vi "initialize.vi"(0 "HGF_IMAQDevice":refnum<class "HGF_ImaqFg.lvclass">, 3 "initializationData":variant, 5 "error in (no error)":errorcluster, 7 "binaryString":string, 8 "I8 Array":i8[](array[numeric]), 9 "prependSize? (T)":bool, 11 "byteOrder (0:big-endian, network order)":T1(ring)) -> (14 "dup HGF_IMAQDevice":refnum<class "HGF_ImaqFg.lvclass">, 17 "found?":bool, 19 "error out":errorcluster)   [LabVIEW 2014, in "HGF_IMAQ.lvlib" / "HGF_ImaqFg.lvclass"]
doc: "This is a dynamic dispatch VI to be implemented by child classes to initialize their attributes.\n\n<B>Recommendation:</B> Use Variant for initialization data."
uses:
  HGF_ImaqFg.lvclass
  HGF_IMAQDevice/HGF_IMAQDevice.lvclass
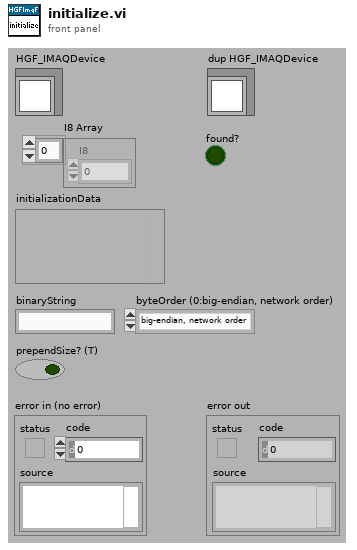
[diagram p1: front panel]
types:
  T1 = enum16{"big-endian, network order", "native, host order", "little-endian"}
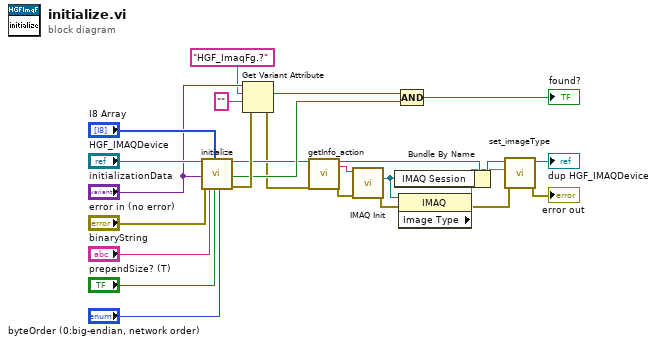
[diagram p0: block diagram]
diagram:
  n1 = call-parent "initialize.vi"("HGF_IMAQDevice"="HGF_IMAQDevice", "initializationData"="initializationData", "error in (no error)"="error in (no error)", "binaryString"="binaryString", "I8 Array"="I8 Array", "prependSize? (T)"="prependSize? (T)", "byteOrder (0:big-endian, network order)"="byteOrder (0:big-endian, network order)") -> ("dup HGF_IMAQDevice"=w12:refnum<class "HGF_ImaqFg.lvclass">, "found?"=w16:bool, "error out"=w18:errorcluster)  [unwired: 10 out]
  n2 = Get Variant Attribute(Variant="initializationData", name="HGF_ImaqFg.?", default value (empty Variant)="", error in=w18) -> (found=w17:bool, error out=w9:errorcluster)  [unwired: 2 out]
  n3 = call-dynamic "getInfo_action.vi"("HGF_ImaqFg"=w12, "error in (no error)"=w9) -> ("dup HGF_ImaqFg"=w11:refnum<class "HGF_ImaqFg.lvclass">, "cameraName"=w8:string, "error out"=w10:errorcluster)  [unwired: 15 out]
  n4 = call <vilib>:"IMAQ Init.vi"("error in (no error)"=w10, "Interface Name"=w8) -> ("error out"=w3:errorcluster, "IMAQ Session Out"=w5:refnum<k11>)  [unwired: 8 out]
  n5 = Bundle By Name(cluster=w11, "IMAQ Session"=w5) -> (w7:refnum<class "HGF_ImaqFg.lvclass">)
  n6 = property class="IMAQ"(reference=w5, error in=w3) -> (error out=w2:errorcluster, "Image Type"=w4)  [unwired: 1 out]
  n7 = Compound Arithmetic op=AND(w17, w16) -> (→"found?":bool)
  n8 = call "set_imageType.vi"("error in (no error)"=w2, "Image Type"=w4, "HGF_IMAQDevice"=w7) -> ("error out"=→"error out":errorcluster, "HGF_IMAQDevice"=→"dup HGF_IMAQDevice":refnum<class "HGF_ImaqFg.lvclass">)  [unwired: 7 out]
